vi "SaveImage.vi"(8 "error in (no error)":errorcluster, 9 "index (-1: latest)":i32=-1, 10 "Path":path, 11 "Camera":refnum<class "Camera.lvclass">) -> (0 "error out":errorcluster, 3 "Camera out":refnum<class "Camera.lvclass">)   [LabVIEW 2015, in "Camera.lvclass"]
doc: "---------------------------------------------------------------\nJKI State Machine Objects™\nhttp://jki.net/state-machine-objects/\nCopyright (C) 2005-2015, JKI <info@jki.net>\nALL RIGHTS RESERVEDJKI State Machine Objects (SMO) 1.0.0.4\nJKI - JKI\nCopyright (c) 2015, JKI"
uses:
  Camera.lvclass
  Camera.lvclass/Camera.ctl
  Typedefs/PrivateEvents--Camera.Save Image.ctl
panel:
  # "For instructions on how to use the JKI State Machine Objects, examples and video tutorials, visit:\nhttp://jki.net/state-machine-objects/\n\nJKI State Machine Objects™\nhttp://jki.net/state-machine-objects/\nCopyright (C) 2005-2015, JKI <info@jki.net>\nALL RIGHTS RESERVED"
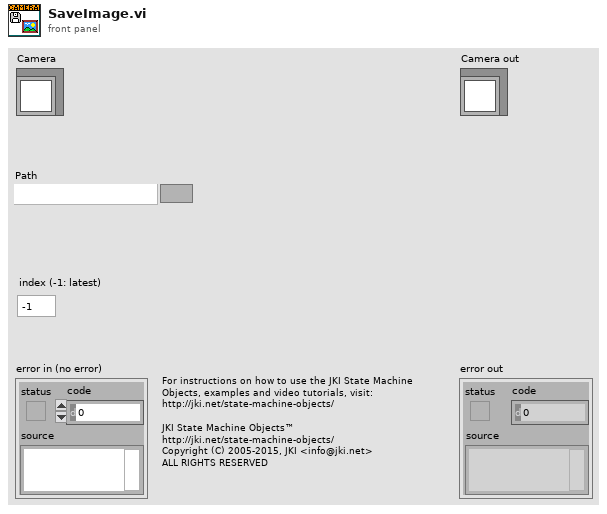
[diagram p1: front panel]
types:
  T1 = typedef "Camera.lvclass/PrivateEvents--Camera.Save Image.ctl" = cluster{"Path":path, "index (-1: latest)":i32}
  T2 = typedef "Camera.lvclass/PrivateData--Ref.ctl" = refnum<data-value>
  T3 = typedef "Camera.lvclass/PrivateData--Cluster.ctl" = cluster{"Public Events":T4, "Protected Events":T5, "Private Events":T6, "Dependencies":T7}
  T4 = typedef "Camera.lvclass/PublicEvents--Cluster.ctl" = cluster{"Value Changed":refnum<user-event>, "NewImage":refnum<user-event>, "ImageSaved":refnum<user-event>}
  T5 = typedef "Camera.lvclass/ProtectedEvents--Cluster.ctl" = cluster{"placeholder":refnum<user-event>}
  T6 = typedef "Camera.lvclass/PrivateEvents--Cluster.ctl" = cluster{"New Value":refnum<user-event>, "Grab Image":refnum<user-event>, "Save Image":refnum<user-event>, "Get Image":refnum<user-event>}
  T7 = typedef "Camera.Simulated.lvclass/Dependencies--Cluster.ctl" = cluster{"CircularBuffer.ImageData":refnum<class "CircularBuffer.ImageData.lvclass">}
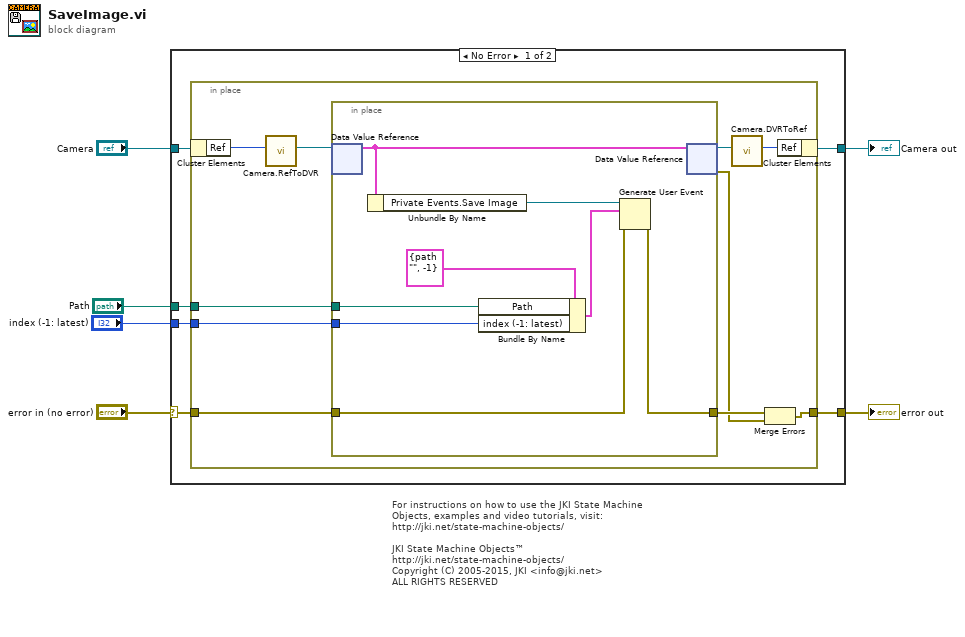
[diagram p0: block diagram]
diagram:
  # "For instructions on how to use the JKI State Machine Objects, examples and video tutorials, visit:\nhttp://jki.net/state-machine-objects/\n\nJKI State Machine Objects™\nhttp://jki.net/state-machine-objects/\nCopyright (C) 2005-2015, JKI <info@jki.net>\nALL RIGHTS RESERVED"
  n1 = case shown="No Error" "error in (no error)" {
    selector: "error in (no error)" -> [w10 w32]
    tunnel: [w9 w32] -> w5
    tunnel: [w11 w31] -> w6
    tunnel: "Camera" -> [w12 w31]
    tunnel: "Path" -> [w8 _]
    tunnel: "index (-1: latest)" -> [w7 _]
    frame No Error {
      n2 = in-place {
        in-place-border: w10 -> [w22]
        in-place-border: [w19] -> w9
        in-place-border: w8 -> [w16]
        in-place-border: w7 -> [w13]
        n3 = in-place-cluster #1(w12) -> ("Ref"=w18:u32)
        n4 = call "Camera.RefToDVR.vi"("Ref"=w18) -> ("Ref"=w15:T2)  [unwired: 10 in]
        n5 = in-place {
          in-place-border: w22 -> [w28]
          in-place-border: [w27] -> w21
          in-place-border: w16 -> [w25]
          in-place-border: w13 -> [w23]
          n6 = in-place-dvr #2(w15) -> (w30:T3)  [unwired: 1 out]
          n7 = Unbundle By Name(w30) -> ("Private Events.Save Image"=w29:refnum<user-event>)
          n8 = Bundle By Name(cluster=T1 {"Path"=path "", "index (-1: latest)"=-1} ("Save Image"), "Path"=w25, "index (-1: latest)"=w23) -> (w24:T1)
          n9 = Generate User Event(user event=w29, event data cluster=w24, error in=w28) -> (error out=w27:errorcluster)  [unwired: 1 in, 1 out]
          n10 = in-place-dvr #2(w30) -> (w17:T2, w20:errorcluster)
        }
        n11 = call "Camera.DVRToRef.vi"("Ref"=w17) -> ("Ref"=w14:u32)  [unwired: 10 in]
        n12 = Merge Errors(w21, w20) -> (w19:errorcluster)
        n13 = in-place-cluster #1("Ref"=w14) -> (w11:refnum<class "Camera.lvclass">)
      }
    }
    frame Error {
    }
  }
  "error out" <- w5
  "Camera out" <- w6
